vi "Negate_Qin_4channel.vi"(8 "valid in":bool, 11 "Data in":fxp<+/-,16,14>[](array[numeric])=[0.0, 0.0, 0.0, 0.0, 0.0, 0.0, 0.0, 0.0]) -> (0 "valid out":bool, 3 "Data out":fxp<+/-,16,14>[](array[numeric]))   [LabVIEW 2013]
uses:
  <vilib>/rvi/FXPMathLib/FxpConvert/subVIs/nifxpmath_Convert_SimConfig.ctl
  <vilib>/fxp/LVFixedPointQuantizationPolicyTypeDef.ctl
  <vilib>/fxp/LVFixedPointOverflowPolicyTypeDef.ctl
  <vilib>/rvi/FXPMathLib/FxpConvert/simVIs/DllFxpConvertTemp_sub.vi
  <vilib>/rvi/FXPMathLib/FxpConvert/XNode/nifxpmath_Convert.xnode
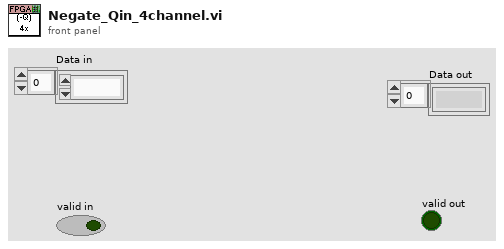
[diagram p1: front panel]
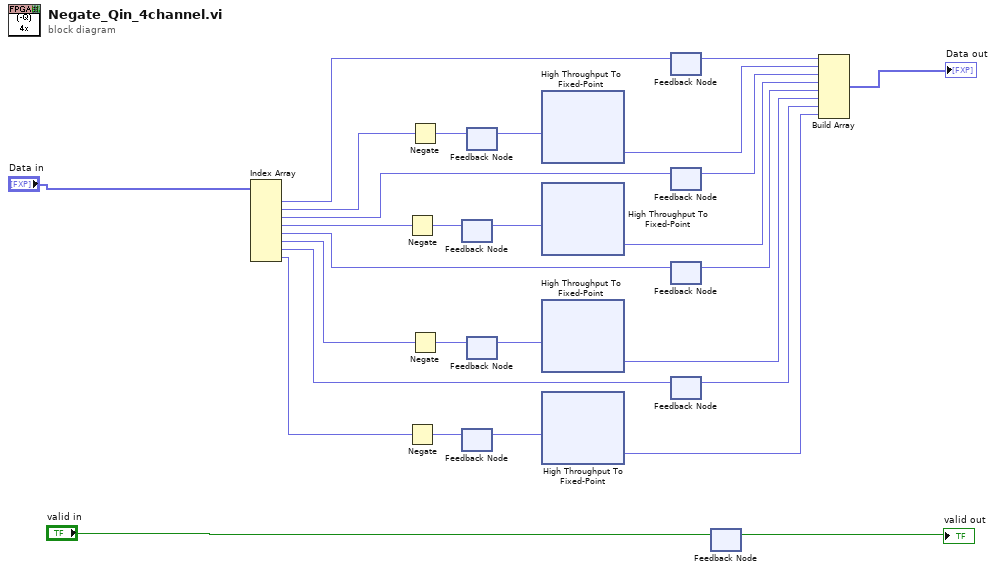
[diagram p0: block diagram]
diagram:
  n1 = Index Array(array="Data in") -> (element #1=w22:fxp<+/-,16,14>, element #2=w21:fxp<+/-,16,14>, element #3=w17:fxp<+/-,16,14>, element #4=w19:fxp<+/-,16,14>, element #5=w8:fxp<+/-,16,14>, element #6=w7:fxp<+/-,16,14>, element #7=w6:fxp<+/-,16,14>, element #8=w5:fxp<+/-,16,14>)  [unwired: 8 in]
  n2 = Negate(x=w19) -> (-x=w18:fxp<+/-,17,15>)
  n3 = Negate(x=w5) -> (-x=w10:fxp<+/-,17,15>)
  n4 = Negate(x=w21) -> (-x=w20:fxp<+/-,17,15>)
  n5 = Negate(x=w7) -> (-x=w9:fxp<+/-,17,15>)
  n6 = feedback #1() -> (w16:fxp<+/-,17,15>)  [unwired: 1 in]
  n7 = feedback-in #1(w18) -> ()
  n8 = feedback #2() -> (w11:fxp<+/-,17,15>)  [unwired: 1 in]
  n9 = feedback-in #2(w10) -> ()
  n10 = feedback #3() -> (w13:fxp<+/-,17,15>)  [unwired: 1 in]
  n11 = feedback-in #3(w20) -> ()
  n12 = feedback #4() -> (w12:fxp<+/-,17,15>)  [unwired: 1 in]
  n13 = feedback-in #4(w9) -> ()
  n14 = xnode "High Throughput To Fixed-Point"("x"=w13) -> ("y"=w14:fxp<+/-,16,14>)
  n15 = xnode "High Throughput To Fixed-Point"("x"=w16) -> ("y"=w15:fxp<+/-,16,14>)
  n16 = xnode "High Throughput To Fixed-Point"("x"=w12) -> ("y"=w3:fxp<+/-,16,14>)
  n17 = xnode "High Throughput To Fixed-Point"("x"=w11) -> ("y"=w1:fxp<+/-,16,14>)
  n18 = feedback #5() -> (w24:fxp<+/-,16,14>)  [unwired: 1 in]
  n19 = feedback-in #5(w22) -> ()
  n20 = feedback #6() -> (w23:fxp<+/-,16,14>)  [unwired: 1 in]
  n21 = feedback-in #6(w17) -> ()
  n22 = feedback #7() -> (w4:fxp<+/-,16,14>)  [unwired: 1 in]
  n23 = feedback-in #7(w8) -> ()
  n24 = feedback #8() -> (w2:fxp<+/-,16,14>)  [unwired: 1 in]
  n25 = feedback-in #8(w6) -> ()
  n26 = feedback #9() -> (→"valid out":bool)  [unwired: 1 in]
  n27 = feedback-in #9("valid in") -> ()
  n28 = Build Array(w24, w14, w23, w15, w4, w3, w2, w1) -> (→"Data out":fxp<+/-,16,14>[])
